vi "SP Perform Filter Skirt Limit Testing.vi"(0 "Filter Limit":T12={"Limit #"=1, "Parameter"={"Stimulus Port"=1, "Response Port"=2}, "Format"=enum."Lin Mag", "Filter Type"=enum."Bandpass", "Passband"={"Start/Center"=510.0, "Stop/Span"=610.0, "Units"=enum."MHz", "Freq Format"=enum."Start/Stop", "Bandwidth Attn"=3.0, "Passband Limit"=FALSE}, "Ripple"={"Ripple Limit"=TRUE, "Window On"=FALSE, "Ripple"=0.1, "Window"=10.0, "Units"=enum."MHz"}, "Attenuation Points"=[], "Skirt Points"=[{"Relative"=TRUE, "Connect"=FALSE, "Frequency"=500.0, "Units"=enum."MHz", "Attenuation"=4.0, "Relative Loss"=enum."Calculated Center", "Relative Freq"=1000.0}, {"Relative"=TRUE, "Connect"=TRUE, "Frequency"=509.0, "Units"=enum."MHz", "Attenuation"=4.0, "Relative Loss"=enum."Calculated Center", "Relative Freq"=1000.0}, {"Relative"=TRUE, "Connect"=FALSE, "Frequency"=611.0, "Units"=enum."MHz", "Attenuation"=4.0, "Relative Loss"=enum."Calculated Center", "Relative Freq"=1000.0}, {"Relative"=TRUE, "Connect"=TRUE, "Frequency"=620.0, "Units"=enum."MHz", "Attenuation"=4.0, "Relative Loss"=enum."Calculated Center", "Relative Freq"=1000.0}]} {"Parameter"."Stimulus Port" min=1 step=1; "Parameter"."Response Port" min=1 step=1; "Passband"."Bandwidth Attn" format="%.3g"; "Passband"."Stop/Span" format="%.3g"; "Passband"."Start/Center" format="%.3g"}, 5 "Data":T11={"F0"=500.0, "dF"=1.0, "Formatted Values"=[-6.0, -6.0, -6.0, -6.0, -6.0, -6.0, -5.0, -4.0, -3.0, -2.0, -1.0017226002993769, -0.8636286738753696, -1.012432061728755, -0.8135188671805874, -1.084383696215112, -1.192695586219516, -0.8228939725524264, -1.1588169801015764, -1.0069715761898415, -0.8118111488159718, -0.9516999033989667, -1.0842662636672022, -1.0261931083967077, -0.816874162233468, -0.8335770068326294, -1.1794529347576463, -1.1032959879886735, -1.197742447623333, -0.9631229100196212, -0.9908453124177325, -0.9835470980893588, -1.10217991844936, -0.8956607286257672, -0.8794782872077156, -0.9013683651609963, -1.0772188731817596, -0.992723355191172, -0.9536275499498994, -0.9874327685983141, -0.921963653527827, -0.8848787728556787, -1.1874980208218, -0.996957511881206, -0.9972503730309241, -0.8866139538542095, -1.07344181331393, -0.881559772443858, -1.0112449407130875, -0.9865384477979471, -0.9901446738263366, -1.1718630063784758, -0.9951725256878827, -0.931778781153855, -0.9846289731021831, -0.851763264124267, -0.9086965469391421, -0.8349429101974368, -0.8383742350256687, -1.106571816484691, -0.9554005266395742, -0.9376822403043366, -1.131287512516927, -1.0382288806403288, -0.917054052988136, -0.9489467877812984, -0.9264227759143271, -1.0918690925892351, -1.1668737446636852, -1.0021735712381068, -1.1541225361979714, -1.1931131329605709, -0.8730502330378824, -0.850411285659811, -1.137775166801135, -1.1870586525662095, -1.0926571181161528, -1.118993526927924, -1.1211410787283602, -0.8920697041785735, -0.888430731015914, -1.0656600076605476, -1.1666787859795846, -1.0713340188424678, -0.8625910088884297, -1.1434360227216422, -0.9217710376784376, -1.1218396445954617, -0.9558195687190933, -1.1773692443654946, -1.0827782751424972, -1.1567791336122029, -0.8684407402614696, -0.8177845157195978, -0.9040657051180614, -0.9313557288389804, -1.0236831450620423, -1.050426714979035, -0.8344777069605718, -0.8274082929927138, -1.1990080831766776, -1.0947798998491134, -1.1963114865246718, -1.0016247375583676, -1.0877110100652403, -1.1556028882288836, -1.1918380581525247, -0.9751292214691399, -0.8884133044813358, -1.0347444321214612, -0.9445125246491541, -2.0, -3.0, -4.0, -5.0, -6.0, -6.0, -6.0, -6.0, -6.0, -6.0]}, 9 "Generate Plot Output? (f)":bool, 11 "error in (no error)":errorcluster, 12 "Limit Results In":T2={"Limit #"=0, "Parameter"={"Stimulus Port"=1, "Response Port"=0}, "Bandwidth Pass?"={"Pass?"=FALSE, "Bandwidth"=0.0, "Limit"=0.0, "Units"=enum."Hz"}, "Ripple Pass?"={"Pass?"=FALSE, "Ripple"=0.0, "Limit"=0.0, "Format"=enum."Log Mag"}, "Attenuation Results"=[], "Skirt Results"=[], "Pass?"=FALSE} {"Parameter"."Stimulus Port" min=1 step=1; "Parameter"."Response Port" min=1 step=1}, 13 "Format":T1 caption="Display Format" items=["Log Mag", "Phase", "Expanded Phase", "Delay", "Smith", "Polar", "Lin Mag", "SWR", "Loss", "Real", "Imaginary"]) -> (1 "Upper Limits":cluster{"x values":dbl[], "y values":dbl[]}[](array[cluster]), 3 "Lower Limits":cluster{"x values":dbl[], "y values":dbl[]}[](array[cluster]), 4 "Limits Pass/Fail":cluster{"Upper Pass?":bool, "Lower Pass?":bool}, 6 "Upper and Lower Limits":T10={"Upper Limit"={"F0"=500.0, "dF"=1.0, "Formatted Values"=[-6.0, -6.0, -6.0, -6.0, -6.0, -6.0, -5.0, -4.0, -3.0, -2.0, -1.0017226002993769, -0.8636286738753696, -1.012432061728755, -0.8135188671805874, -1.084383696215112, -1.192695586219516, -0.8228939725524264, -1.1588169801015764, -1.0069715761898415, -0.8118111488159718, -0.9516999033989667, -1.0842662636672022, -1.0261931083967077, -0.816874162233468, -0.8335770068326294, -1.1794529347576463, -1.1032959879886735, -1.197742447623333, -0.9631229100196212, -0.9908453124177325, -0.9835470980893588, -1.10217991844936, -0.8956607286257672, -0.8794782872077156, -0.9013683651609963, -1.0772188731817596, -0.992723355191172, -0.9536275499498994, -0.9874327685983141, -0.921963653527827, -0.8848787728556787, -1.1874980208218, -0.996957511881206, -0.9972503730309241, -0.8866139538542095, -1.07344181331393, -0.881559772443858, -1.0112449407130875, -0.9865384477979471, -0.9901446738263366, -1.1718630063784758, -0.9951725256878827, -0.931778781153855, -0.9846289731021831, -0.851763264124267, -0.9086965469391421, -0.8349429101974368, -0.8383742350256687, -1.106571816484691, -0.9554005266395742, -0.9376822403043366, -1.131287512516927, -1.0382288806403288, -0.917054052988136, -0.9489467877812984, -0.9264227759143271, -1.0918690925892351, -1.1668737446636852, -1.0021735712381068, -1.1541225361979714, -1.1931131329605709, -0.8730502330378824, -0.850411285659811, -1.137775166801135, -1.1870586525662095, -1.0926571181161528, -1.118993526927924, -1.1211410787283602, -0.8920697041785735, -0.888430731015914, -1.0656600076605476, -1.1666787859795846, -1.0713340188424678, -0.8625910088884297, -1.1434360227216422, -0.9217710376784376, -1.1218396445954617, -0.9558195687190933, -1.1773692443654946, -1.0827782751424972, -1.1567791336122029, -0.8684407402614696, -0.8177845157195978, -0.9040657051180614, -0.9313557288389804, -1.0236831450620423, -1.050426714979035, -0.8344777069605718, -0.8274082929927138, -1.1990080831766776, -1.0947798998491134, -1.1963114865246718, -1.0016247375583676, -1.0877110100652403, -1.1556028882288836, -1.1918380581525247, -0.9751292214691399, -0.8884133044813358, -1.0347444321214612, -0.9445125246491541, -2.0, -3.0, -4.0, -5.0, -6.0, -6.0, -6.0, -6.0, -6.0, -6.0]}, "Lower Limit"={"F0"=500.0, "dF"=1.0, "Formatted Values"=[-6.0, -6.0, -6.0, -6.0, -6.0, -6.0, -5.0, -4.0, -3.0, -2.0, -1.0017226002993769, -0.8636286738753696, -1.012432061728755, -0.8135188671805874, -1.084383696215112, -1.192695586219516, -0.8228939725524264, -1.1588169801015764, -1.0069715761898415, -0.8118111488159718, -0.9516999033989667, -1.0842662636672022, -1.0261931083967077, -0.816874162233468, -0.8335770068326294, -1.1794529347576463, -1.1032959879886735, -1.197742447623333, -0.9631229100196212, -0.9908453124177325, -0.9835470980893588, -1.10217991844936, -0.8956607286257672, -0.8794782872077156, -0.9013683651609963, -1.0772188731817596, -0.992723355191172, -0.9536275499498994, -0.9874327685983141, -0.921963653527827, -0.8848787728556787, -1.1874980208218, -0.996957511881206, -0.9972503730309241, -0.8866139538542095, -1.07344181331393, -0.881559772443858, -1.0112449407130875, -0.9865384477979471, -0.9901446738263366, -1.1718630063784758, -0.9951725256878827, -0.931778781153855, -0.9846289731021831, -0.851763264124267, -0.9086965469391421, -0.8349429101974368, -0.8383742350256687, -1.106571816484691, -0.9554005266395742, -0.9376822403043366, -1.131287512516927, -1.0382288806403288, -0.917054052988136, -0.9489467877812984, -0.9264227759143271, -1.0918690925892351, -1.1668737446636852, -1.0021735712381068, -1.1541225361979714, -1.1931131329605709, -0.8730502330378824, -0.850411285659811, -1.137775166801135, -1.1870586525662095, -1.0926571181161528, -1.118993526927924, -1.1211410787283602, -0.8920697041785735, -0.888430731015914, -1.0656600076605476, -1.1666787859795846, -1.0713340188424678, -0.8625910088884297, -1.1434360227216422, -0.9217710376784376, -1.1218396445954617, -0.9558195687190933, -1.1773692443654946, -1.0827782751424972, -1.1567791336122029, -0.8684407402614696, -0.8177845157195978, -0.9040657051180614, -0.9313557288389804, -1.0236831450620423, -1.050426714979035, -0.8344777069605718, -0.8274082929927138, -1.1990080831766776, -1.0947798998491134, -1.1963114865246718, -1.0016247375583676, -1.0877110100652403, -1.1556028882288836, -1.1918380581525247, -0.9751292214691399, -0.8884133044813358, -1.0347444321214612, -0.9445125246491541, -2.0, -3.0, -4.0, -5.0, -6.0, -6.0, -6.0, -6.0, -6.0, -6.0]}}, 10 "Failures":cluster{"x values":dbl[], "y values":dbl[]}[](array[cluster]), 14 "Limit Results Out":T2={"Limit #"=0, "Parameter"={"Stimulus Port"=1, "Response Port"=0}, "Bandwidth Pass?"={"Pass?"=FALSE, "Bandwidth"=0.0, "Limit"=0.0, "Units"=enum."Hz"}, "Ripple Pass?"={"Pass?"=FALSE, "Ripple"=0.0, "Limit"=0.0, "Format"=enum."Log Mag"}, "Attenuation Results"=[], "Skirt Results"=[], "Pass?"=FALSE} {"Parameter"."Stimulus Port" min=1 step=1; "Parameter"."Response Port" min=1 step=1}, 15 "error out":errorcluster)   [LabVIEW 2011]
uses:
  TypeDefs/SP Filter.ctl
  TypeDefs/SP Parameter.ctl
  TypeDefs/SP Format.ctl
  TypeDefs/SP Filter Type.ctl
  TypeDefs/SP Filter Passband.ctl
  TypeDefs/SP Frequency Units.ctl
  TypeDefs/SP Frequency Format.ctl
  TypeDefs/SP Filter Ripple.ctl
  TypeDefs/SP Attenuation Point.ctl
  TypeDefs/SP Attenuation Type.ctl
  TypeDefs/SP Skirt Rejection Point.ctl
  TypeDefs/SP Relative Loss.ctl
  TypeDefs/SP Limit Results.ctl
  TypeDefs/SP Bandwidth Limit Results.ctl
  TypeDefs/SP Ripple Limit Results.ctl
  TypeDefs/SP Attenuation Limit Results.ctl
  TypeDefs/SP Skirt Limit Results.ctl
  TypeDefs/SP Display Format.ctl
  <vilib>/Analysis/NI_AALBase.lvlib
panel:
  out "Plot Output":cluster{"x values":dbl[], "y values":dbl[]}[](graph)
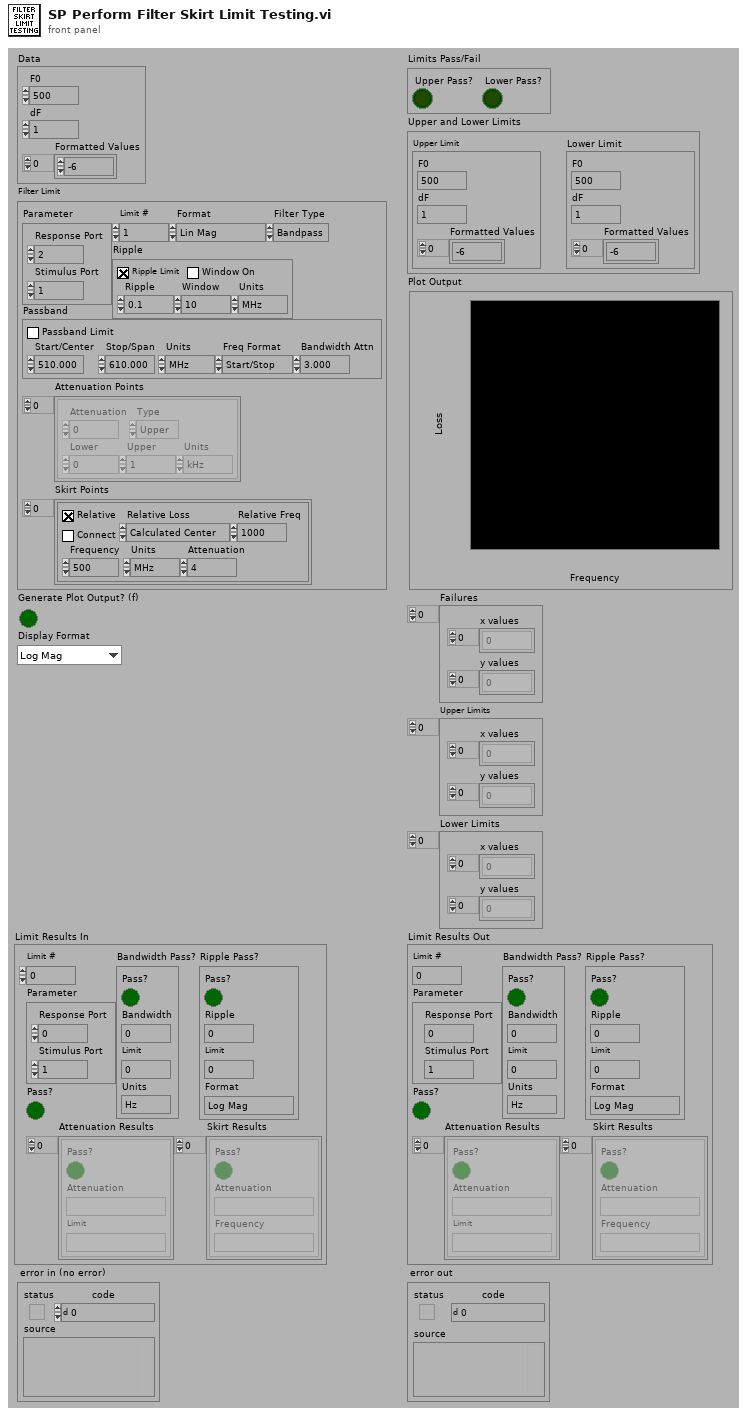
[diagram p1: front panel]
types:
  T1 = typedef "SP Display Format.ctl" = i32
  T2 = typedef "SP Limit Results.ctl" = cluster{"Limit #":i8, "Parameter":T3, "Bandwidth Pass?":T4, "Ripple Pass?":T6, "Attenuation Results":T8[], "Skirt Results":T9[], "Pass?":bool}
  T3 = typedef "SP Parameter.ctl" = cluster{"Stimulus Port":i8, "Response Port":i8}
  T4 = typedef "SP Bandwidth Limit Results.ctl" = cluster{"Pass?":bool, "Bandwidth":dbl, "Limit":dbl, "Units":T5}
  T5 = typedef "SP Frequency Units.ctl" = enum16{"Hz", "kHz", "MHz", "GHz", "Points"}
  T6 = typedef "SP Ripple Limit Results.ctl" = cluster{"Pass?":bool, "Ripple":dbl, "Limit":dbl, "Format":T7}
  T7 = typedef "SP Format.ctl" = enum16{"Log Mag", "Lin Mag", "SWR", "Phase", "Expanded Phase", "Delay", "Insertion Loss", "Isolation", "Return Loss"}
  T8 = typedef "SP Attenuation Limit Results.ctl" = cluster{"Pass?":bool, "Attenuation":string, "Limit":string}
  T9 = typedef "SP Skirt Limit Results.ctl" = cluster{"Pass?":bool, "Attenuation":string, "Frequency":string}
  T10 = cluster{"Upper Limit":cluster{"F0":dbl, "dF":dbl, "Formatted Values":dbl[]}, "Lower Limit":cluster{"F0":dbl, "dF":dbl, "Formatted Values":dbl[]}}
  T11 = cluster{"F0":dbl, "dF":dbl, "Formatted Values":dbl[]}
  T12 = typedef "SP Filter.ctl" = cluster{"Limit #":i8, "Parameter":T3, "Format":T7, "Filter Type":T13, "Passband":T14, "Ripple":T16, "Attenuation Points":T17[], "Skirt Points":T19[]}
  T13 = typedef "SP Filter Type.ctl" = enum16{"Lowpass", "Highpass", "Bandpass", "Bandstop"}
  T14 = typedef "SP Filter Passband.ctl" = cluster{"Start/Center":dbl, "Stop/Span":dbl, "Units":T5, "Freq Format":T15, "Bandwidth Attn":dbl, "Passband Limit":bool}
  T15 = typedef "SP Frequency Format.ctl" = enum16{"Start/Stop", "Center/Span"}
  T16 = typedef "SP Filter Ripple.ctl" = cluster{"Ripple Limit":bool, "Window On":bool, "Ripple":dbl, "Window":dbl, "Units":T5}
  T17 = typedef "SP Attenuation Point.ctl" = cluster{"Attenuation":dbl, "Type":T18, "Lower":dbl, "Upper":dbl, "Units":T5}
  T18 = typedef "SP Attenuation Type.ctl" = enum16{"Center", "Lower", "Upper"}
  T19 = typedef "SP Skirt Rejection Point.ctl" = cluster{"Relative":bool, "Connect":bool, "Frequency":dbl, "Units":T5, "Attenuation":dbl, "Relative Loss":T20, "Relative Freq":dbl}
  T20 = typedef "SP Relative Loss.ctl" = enum16{"Calculated Center", "Passband Minimum", "Passband Maximum", "Passband Average", "Frequency"}
  T21 = cluster{"x0":dbl, "dx":dbl, "Stored Values":dbl[]}
  T22 = cluster{"Limit":cluster{"x0":dbl, "dx":dbl, "Y":dbl[]}, "Limit":cluster{"x0":dbl, "dx":dbl, "Stored Values":dbl[]}}
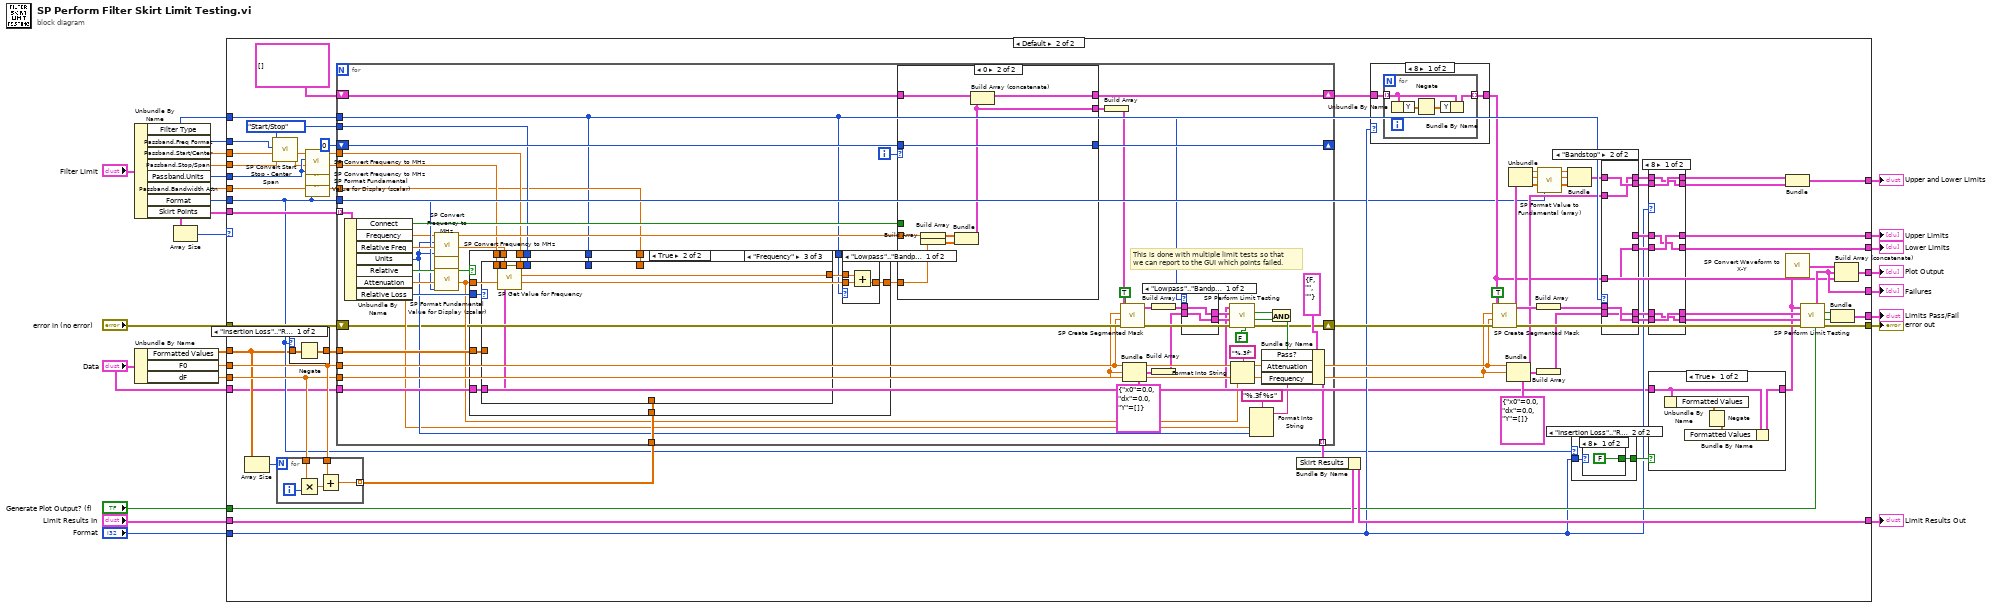
[diagram p0: block diagram]
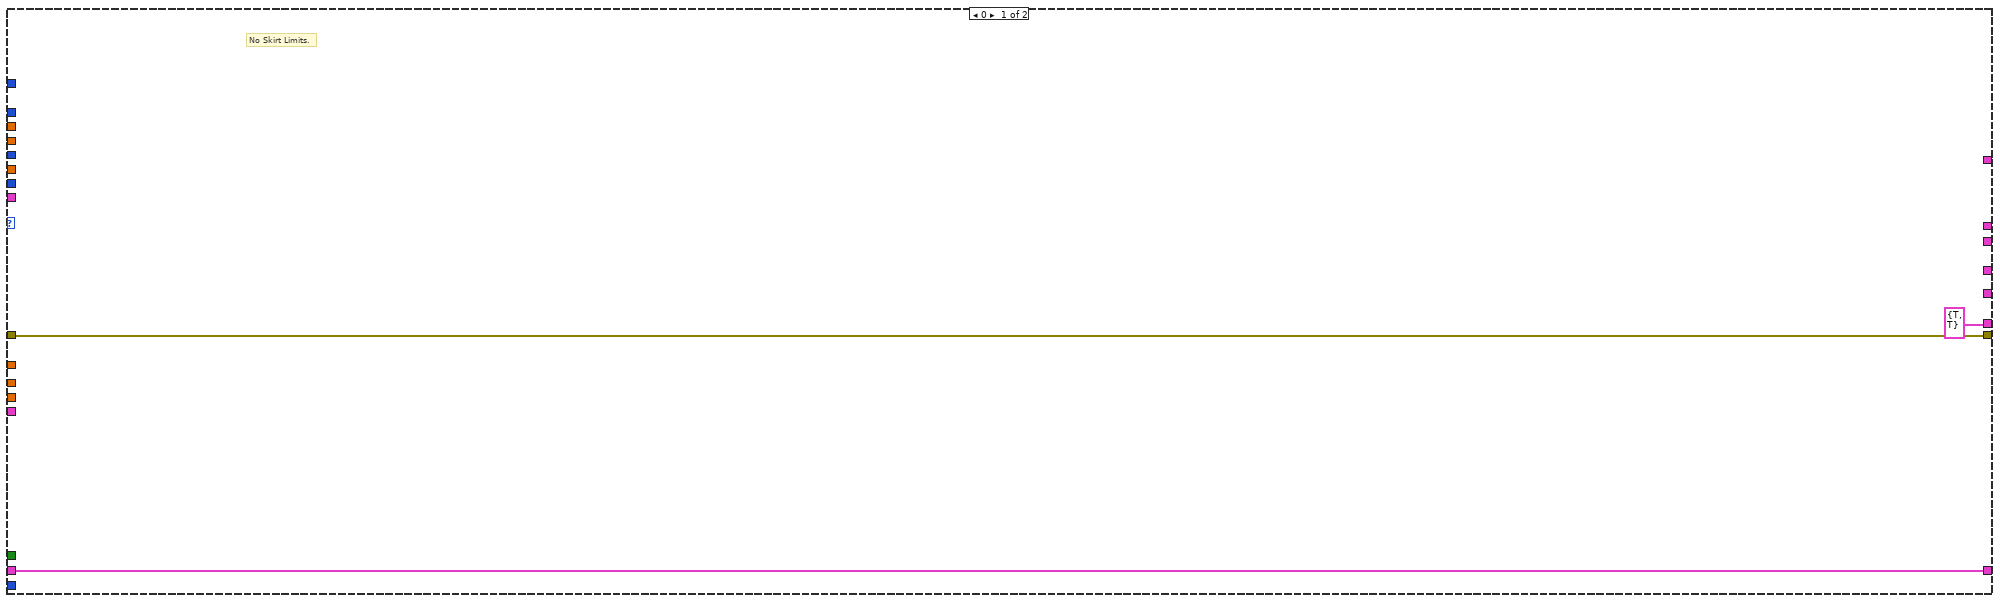
[diagram p2: hidden frame]
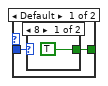
[diagram p4: hidden frame]
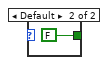
[diagram p5: hidden frame]
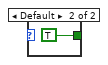
[diagram p6: hidden frame]
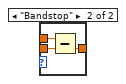
[diagram p13: hidden frame]
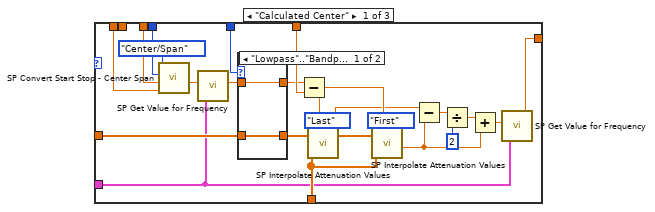
[diagram p14: hidden frame]
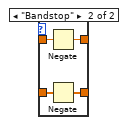
[diagram p15: hidden frame]
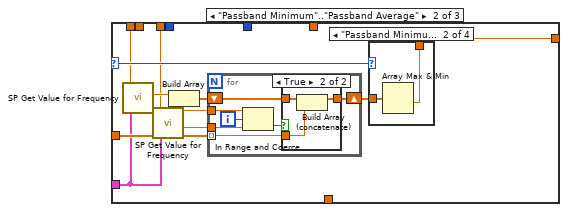
[diagram p16: hidden frame]
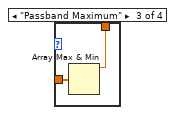
[diagram p18: hidden frame]
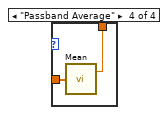
[diagram p19: hidden frame]
diagram:
  n1 = Unbundle By Name("Filter Limit") -> ("Filter Type"=w17:T13, "Passband.Freq Format"=w16:T15, "Passband.Start/Center"=w25:dbl, "Passband.Stop/Span"=w24:dbl, "Passband.Units"=w23:T5, "Passband.Bandwidth Attn"=w12:dbl, "Format"=w13:T7, "Skirt Points"=w14:T19[])
  n2 = Unbundle By Name("Data") -> ("Formatted Values"=w22:dbl[], "F0"=w11:dbl, "dF"=w10:dbl)
  n3 = Array Size(array=w14) -> (size(s)=w15:i32)
  n4 = case shown="Default" w15 {
    tunnel: w17 -> [_ w76]
    tunnel: w25 -> [_ w90]
    tunnel: w24 -> [_ w89]
    tunnel: w23 -> [_ w95]
    tunnel: w22 -> [_ w32]
    tunnel: "Data" -> [_ w31]
    tunnel: "Generate Plot Output? (f)" -> [_ w67]
    tunnel: "error in (no error)" -> [w29 w71]
    tunnel: [w29 w92] -> w18
    tunnel: w16 -> [_ w86]
    tunnel: w14 -> [_ w85]
    tunnel: w13 -> [_ w33]
    tunnel: w12 -> [_ w82]
    tunnel: w11 -> [_ w64]
    tunnel: w10 -> [_ w63]
    tunnel: [_ w74] -> w9
    tunnel: [_ w66] -> w8
    tunnel: [_ w37] -> w7
    tunnel: [_ w30] -> w6
    tunnel: "Limit Results In" -> [w28 w70]
    tunnel: [w28 w69] -> w4
    tunnel: [cluster{"Upper Pass?":bool, "Lower Pass?":bool} {"Upper Pass?"=TRUE, "Lower Pass?"=TRUE} w59] -> w3
    tunnel: [_ w51] -> w2
    tunnel: "Format" -> [_ w34]
    frame 0 {
      # "No Skirt Limits."
    }
    frame Default {
      w83 = SP_Frequency_Format."Start/Stop" ("Freq Format To")
      n5 = Array Size(array=w32) -> (size(s)=w80:i32)
      n6 = call "SP Convert Start Stop - Center Span.vi"("Stop/Span In"=w89, "Start/Center In"=w90, "Freq Format From"=w86, "Freq Format To"=w83) -> ("Stop/Span Out"=w88:dbl, "Start/Center Out"=w87:dbl)  [unwired: 6 out]
      n7 = for {
        N: w80 -> [_]
        tunnel: w63 -> [w144]
        tunnel: w64 -> [w142]
        tunnel: [w141] -> w79 mode=indexing
        i -> [w145]
        n8 = Multiply(x=w144, y=w145) -> (x*y=w143:dbl)
        n9 = Add(x=w142, y=w143) -> (x+y=w141:dbl)
      }
      n10 = case shown="\"Insertion Loss\"..\"Return Loss\"" w33 {
        tunnel: w32 -> [w129 w130]
        tunnel: [w128 w130] -> w50
        frame "Insertion Loss".."Return Loss" {
          n11 = Negate(x=w129) -> (-x=w128:dbl[])
        }
        frame Default {
        }
      }
      n12 = call "SP Convert Frequency to MHz.vi"("Units"=w95, "Frequency"=w87) -> ("Converted Frequency"=w93:dbl)  [unwired: 1 in, 8 out]
      n13 = call "SP Convert Frequency to MHz.vi"("Units"=w95, "Frequency"=w88) -> ("Converted Frequency"=w94:dbl)  [unwired: 1 in, 8 out]
      n14 = call "SP Format Fundamental Value for Display (scalar).vi"("Format"=w33, "Stored Value (0, linear)"=w82) -> ("Display Value"=w81:dbl)  [unwired: 5 out]
      n15 = for {
        tunnel: w94 -> [w181]
        tunnel: w93 -> [w182]
        tunnel: w85 -> [w196] mode=indexing
        shift-right: [w193] -> w49
        shift-left: cluster{"X":dbl[], "Y":dbl[]}[] [] ("Limit Specification") -> [w194]
        shift-right: [w192] -> _
        shift-left: 0 -> [w191]
        tunnel: w33 -> [w184]
        tunnel: w83 -> [w179]
        tunnel: w81 -> [w178]
        tunnel: w76 -> [w155]
        tunnel: w50 -> [w177]
        tunnel: w31 -> [w156]
        tunnel: w79 -> [w176]
        shift-right: [w151] -> w72
        shift-left: w71 -> [w158]
        tunnel: w64 -> [w149]
        tunnel: w63 -> [w148]
        tunnel: [w174] -> w68 mode=indexing
        i -> [w195]
        # "This is done with multiple limit tests so that\nwe can report to the GUI which points failed."
        n16 = Unbundle By Name(w196) -> ("Connect"=w188:bool, "Frequency"=w169:dbl, "Relative Freq"=w189:dbl, "Units"=w170:T5, "Relative"=w186:bool, "Attenuation"=w187:dbl, "Relative Loss"=w183:T20)
        n17 = call "SP Convert Frequency to MHz.vi"("Units"=w170, "Frequency"=w169) -> ("Converted Frequency"=w190:dbl)  [unwired: 1 in, 8 out]
        n18 = call "SP Convert Frequency to MHz.vi"("Units"=w170, "Frequency"=w189) -> ("Converted Frequency"=w180:dbl)  [unwired: 1 in, 8 out]
        n19 = call "SP Format Fundamental Value for Display (scalar).vi"("Format"=w184, "Stored Value (0, linear)"=w187) -> ("Display Value"=w172:dbl)  [unwired: 5 out]
        n20 = case shown="True" w186 {
          tunnel: w172 -> [w201 w209]
          tunnel: [w201 w208] -> w185
          tunnel: w183 -> [_ w215]
          tunnel: w182 -> [_ w214]
          tunnel: w181 -> [_ w213]
          tunnel: w177 -> [_ w212]
          tunnel: w180 -> [_ w211]
          tunnel: w179 -> [_ w207]
          tunnel: w156 -> [_ w206]
          tunnel: w155 -> [_ w205]
          tunnel: w178 -> [_ w204]
          tunnel: w176 -> [_ w203]
          tunnel: w155 -> [_ w202]
          frame False {
          }
          frame True {
            n21 = case shown="\"Frequency\"" w215 {
              selector: w215 -> [_ w258 _]
              tunnel: w214 -> [w242 w254 _]
              tunnel: w213 -> [w243 w256 _]
              tunnel: w212 -> [w232 w261 _]
              tunnel: [w224 w259 w281] -> w210
              tunnel: w211 -> [_ _ w282]
              tunnel: w207 -> [w241 _ _]
              tunnel: w206 -> [w226 w251 w280]
              tunnel: w205 -> [w234 _ _]
              tunnel: w204 -> [w223 _ _]
              tunnel: w203 -> [w239 _ _]
              frame "Calculated Center" {
                n22 = call "SP Convert Start Stop - Center Span.vi"("Stop/Span In"=w243, "Start/Center In"=w242, "Freq Format From"=w241, "Freq Format To"=SP_Frequency_Format."Center/Span") -> ("Start/Center Out"=w240:dbl)  [unwired: 7 out]
                n23 = call "SP Get Value for Frequency.vi"("Data"=w226, "Frequency (MHz)"=w240) -> ("Value"=w233:dbl)  [unwired: 5 out]
                n24 = case shown="\"Lowpass\"..\"Bandpass\"" w234 {
                  tunnel: w233 -> [w245 w250]
                  tunnel: w232 -> [w246 w248]
                  tunnel: [w246 w247] -> w231
                  tunnel: [w245 w249] -> w222
                  frame "Lowpass".."Bandpass" {
                  }
                  frame "Bandstop" {
                    n25 = Negate(x=w250) -> (-x=w249:dbl)
                    n26 = Negate(x=w248) -> (-x=w247:dbl[])
                  }
                }
                n27 = Subtract(x=w222, y=w223) -> (x-y=w236:dbl)
                n28 = call "SP Interpolate Attenuation Values.vi"("Instance (First)"=enum16{"First", "Last"}."Last", "Attenuation Value"=w236, "X Values"=w239, "Y Values"=w231) -> ("Interpolated X Value"=w235:dbl)  [unwired: 7 out]
                n29 = call "SP Interpolate Attenuation Values.vi"("Instance (First)"=enum16{"First", "Last"}."First", "Attenuation Value"=w236, "X Values"=w239, "Y Values"=w231) -> ("Interpolated X Value"=w227:dbl)  [unwired: 7 out]
                n30 = Subtract(x=w235, y=w227) -> (x-y=w229:dbl)
                n31 = Divide(x=w229, y=i8 2) -> (x/y=w230:dbl)
                n32 = Add(x=w230, y=w227) -> (x+y=w225:dbl)
                n33 = call "SP Get Value for Frequency.vi"("Data"=w226, "Frequency (MHz)"=w225) -> ("Value"=w224:dbl)  [unwired: 5 out]
              }
              frame "Passband Minimum".."Passband Average" {
                n34 = call "SP Get Value for Frequency.vi"("Data"=w251, "Frequency (MHz)"=w256) -> ("Fractional Index"=w255:dbl, "Value"=w257:dbl)  [unwired: 4 out]
                n35 = call "SP Get Value for Frequency.vi"("Data"=w251, "Frequency (MHz)"=w254) -> ("Fractional Index"=w252:dbl, "Value"=w253:dbl)  [unwired: 4 out]
                n36 = Build Array(w257, w253) -> (w262:dbl[])
                n37 = for {
                  shift-right: [w271] -> w260
                  shift-left: w262 -> [w275]
                  tunnel: w261 -> [w272] mode=indexing
                  tunnel: w255 -> [w270]
                  tunnel: w252 -> [w269]
                  i -> [w274]
                  n38 = In Range and Coerce(upper limit=w270, x=w274, lower limit=w269) -> (In Range?=w273:bool)  [unwired: 1 out]
                  n39 = case shown="True" w273 {
                    tunnel: w275 -> [w276 w279]
                    tunnel: w272 -> [_ w278]
                    tunnel: [w276 w277] -> w271
                    frame False {
                    }
                    frame True {
                      n40 = Build Array (concatenate)(w279, w278) -> (w277:dbl[])
                    }
                  }
                }
                n41 = case shown="\"Passband Minimum\"" w258 {
                  tunnel: w260 -> [_ w264 w266 w268]
                  tunnel: [_ w263 w265 w267] -> w259
                  frame Default {
                  }
                  frame "Passband Minimum" {
                    n42 = Array Max & Min(array=w264) -> (min value=w263:dbl)  [unwired: 3 out]
                  }
                  frame "Passband Maximum" {
                    n43 = Array Max & Min(array=w266) -> (max value=w265:dbl)  [unwired: 3 out]
                  }
                  frame "Passband Average" {
                    n44 = call <vilib>:"Mean.vi"("X"=w268) -> ("mean"=w267:dbl)  [unwired: 1 out]
                  }
                }
              }
              frame "Frequency" {
                n45 = call "SP Get Value for Frequency.vi"("Data"=w280, "Frequency (MHz)"=w282) -> ("Value"=w281:dbl)  [unwired: 5 out]
              }
            }
            n46 = case shown="\"Lowpass\"..\"Bandpass\"" w202 {
              tunnel: w210 -> [w218 w221]
              tunnel: w209 -> [w217 w220]
              tunnel: [w216 w219] -> w208
              frame "Lowpass".."Bandpass" {
                n47 = Add(x=w218, y=w217) -> (x+y=w216:dbl)
              }
              frame "Bandstop" {
                n48 = Subtract(x=w221, y=w220) -> (x-y=w219:dbl)
              }
            }
          }
        }
        n49 = case shown="0" w195 {
          tunnel: w194 -> [w290 w318]
          tunnel: [w289 w317] -> w193
          tunnel: [w287 w312] -> w192
          tunnel: w191 -> [w288 w312]
          tunnel: w190 -> [w285 w316]
          tunnel: w188 -> [w286 _]
          tunnel: w185 -> [w284 w315]
          tunnel: [w283 w311] -> w154
          frame Default {
            n50 = case shown="False" w286 {
              tunnel: w285 -> [w295 w307]
              tunnel: w284 -> [w292 w306]
              tunnel: w288 -> [w297 w302]
              tunnel: w290 -> [w299 w303]
              tunnel: [w296 w302] -> w287
              tunnel: [w298 w301] -> w289
              tunnel: [w291 w300] -> w283
              frame False {
                # "Start a new limit segment..."
                n51 = Build Array(w295) -> (w294:dbl[])
                n52 = Build Array(w292) -> (w293:dbl[])
                n53 = Increment(x=w297) -> (x+1=w296:i32)
                n54 = Bundle(w294, w293) -> (w291:cluster{dbl[], dbl[]})  [unwired: 1 out]
                n55 = Build Array (concatenate)(w299, w291) -> (w298:cluster{"X":dbl[], "Y":dbl[]}[])
              }
              frame True {
                n56 = Index Array(array=w303, index=w302) -> (element=w310:cluster{"X":dbl[], "Y":dbl[]})
                n57 = Unbundle(w310) -> ("X"=w309:dbl[], "Y"=w308:dbl[])
                n58 = Build Array (concatenate)(w309, w307) -> (w305:dbl[])
                n59 = Build Array (concatenate)(w308, w306) -> (w304:dbl[])
                n60 = Bundle(w305, w304) -> (w300:cluster{dbl[], dbl[]})  [unwired: 1 out]
                n61 = Replace Array Subset(array=w303, new element=w300, index=w302) -> (w301:cluster{"X":dbl[], "Y":dbl[]}[])
              }
            }
          }
          frame 0 {
            n62 = Build Array(w316) -> (w314:dbl[])
            n63 = Build Array(w315) -> (w313:dbl[])
            n64 = Bundle(w314, w313) -> (w311:cluster{dbl[], dbl[]})  [unwired: 1 out]
            n65 = Build Array (concatenate)(w318, w311) -> (w317:cluster{"X":dbl[], "Y":dbl[]}[])
          }
        }
        n66 = Build Array(w154) -> (w153:cluster{dbl[], dbl[]}[])
        n67 = call "SP Create Segmented Mask.vi"("Reset"=TRUE, "error in"=w158, "x0"=w149, "dx"=w148, "Specification Cluster"=w153) -> ("error out"=w162:errorcluster, "Limit"=w159:cluster{"x0":dbl, "dx":dbl, "Y":dbl[]})  [unwired: 3 out]
        n68 = Bundle(cluster=cluster{"x0":dbl, "dx":dbl, "Y":dbl[]} {"x0"=0.0, "dx"=0.0, "Y"=[]} ("Limit"), "x0"=w149, "dx"=w148) -> (w147:cluster{"x0":dbl, "dx":dbl, "Y":dbl[]})  [unwired: 1 out]
        n69 = Build Array(w159) -> (w161:cluster{"x0":dbl, "dx":dbl, "Y":dbl[]}[])
        n70 = Build Array(w147) -> (w146:cluster{"x0":dbl, "dx":dbl, "Y":dbl[]}[])
        n71 = case shown="\"Lowpass\"..\"Bandpass\"" w155 {
          tunnel: w161 -> [w198 w200]
          tunnel: [w198 w199] -> w163
          tunnel: [w197 w200] -> w164
          tunnel: w146 -> [w197 w199]
          frame "Lowpass".."Bandpass" {
          }
          frame "Bandstop" {
          }
        }
        n72 = call "SP Perform Limit Testing.vi"("Generate Plot Output? (f)"=FALSE, "error in (no error)"=w162, "LLimits"=w164, "ULimits"=w163, "Data"=w156) -> ("error out"=w151:errorcluster, "Lower Pass?"=w166:bool, "Upper Pass?"=w165:bool)  [unwired: 2 in, 2 out]
        n73 = Format Into String(format string="%.3f", w172) -> (resulting string=w168:string)  [unwired: 2 in, 1 out]
        n74 = Format Into String(format string="%.3f %s", w169, w170) -> (resulting string=w167:string)  [unwired: 2 in, 1 out]
        n75 = And(x=w165, y=w166) -> (x .and. y?=w157:bool)
        n76 = Bundle By Name(cluster=T9 {"Pass?"=FALSE, "Attenuation"="", "Frequency"=""} ("Skirt Results"), "Pass?"=w157, "Attenuation"=w168, "Frequency"=w167) -> (w174:T9)
      }
      n77 = Bundle By Name(cluster=w70, "Skirt Results"=w68) -> (w69:T2)
      n78 = case shown="8" w34 {
        tunnel: w49 -> [w122 w127]
        tunnel: [w121 w127] -> w48
        frame 8 {
          n79 = for {
            tunnel: w122 -> [w126] mode=indexing
            tunnel: [w125] -> w121 mode=indexing
            n80 = Unbundle By Name(w126) -> ("Y"=w124:dbl[])
            n81 = Negate(x=w124) -> (-x=w123:dbl[])
            n82 = Bundle By Name(cluster=w126, "Y"=w123) -> (w125:cluster{"X":dbl[], "Y":dbl[]})
          }
        }
        frame Default {
        }
      }
      n83 = call "SP Create Segmented Mask.vi"("Reset"=TRUE, "error in"=w72, "x0"=w64, "dx"=w63, "Specification Cluster"=w48) -> ("error out"=w78:errorcluster, "Limit"=w54:cluster{"x0":dbl, "dx":dbl, "Y":dbl[]})  [unwired: 3 out]
      n84 = Bundle(cluster=cluster{"x0":dbl, "dx":dbl, "Y":dbl[]} {"x0"=0.0, "dx"=0.0, "Y"=[]} ("Limit"), "x0"=w64, "dx"=w63) -> (w52:cluster{"x0":dbl, "dx":dbl, "Y":dbl[]})  [unwired: 1 out]
      n85 = Unbundle(w54) -> ("x0"=w58:dbl, "dx"=w57:dbl, "Y"=w56:dbl[])
      n86 = Build Array(w54) -> (w77:cluster{"x0":dbl, "dx":dbl, "Y":dbl[]}[])
      n87 = Build Array(w52) -> (w62:cluster{"x0":dbl, "dx":dbl, "Y":dbl[]}[])
      n88 = call "SP Format Value to Fundamental (array).vi"("Sxx Display Format"=w33, "Display Values"=w56) -> ("Stored Values"=w55:dbl[])  [unwired: 5 out]
      n89 = Bundle("x0"=w58, "dx"=w57, "Stored Values"=w55) -> (w53:T21)  [unwired: 1 out]
      n90 = case shown="\"Insertion Loss\"..\"Return Loss\"" w33 {
        tunnel: [w102 w106] -> w36
        tunnel: w34 -> [w101 w105]
        frame Default {
          n91 = case shown="8" w101 {
            tunnel: [TRUE FALSE] -> w102
            frame 8 {
            }
            frame Default {
            }
          }
        }
        frame "Insertion Loss".."Return Loss" {
          n92 = case shown="8" w105 {
            tunnel: [FALSE TRUE] -> w106
            frame 8 {
            }
            frame Default {
            }
          }
        }
      }
      n93 = case shown="\"Bandstop\"" w76 {
        tunnel: w77 -> [w135 w140]
        tunnel: [w135 w138] -> w47
        tunnel: [w133 w140] -> w46
        tunnel: w48 -> [w134 w139]
        tunnel: [_ w139] -> w44
        tunnel: [w134 _] -> w45
        tunnel: w62 -> [w133 w138]
        tunnel: w53 -> [w132 w137]
        tunnel: [w132 w136] -> w42
        tunnel: [w131 w137] -> w43
        tunnel: w52 -> [w131 w136]
        frame "Lowpass".."Bandpass" {
        }
        frame "Bandstop" {
        }
      }
      n94 = case shown="8" w34 {
        tunnel: w47 -> [w110 w117]
        tunnel: w46 -> [w111 w118]
        tunnel: w45 -> [w109 w115]
        tunnel: w44 -> [w112 w116]
        tunnel: w43 -> [w114 w120]
        tunnel: w42 -> [w113 w119]
        tunnel: [w113 w120] -> w41
        tunnel: [w114 w119] -> w40
        tunnel: [w110 w118] -> w39
        tunnel: [w111 w117] -> w38
        tunnel: [w109 w116] -> w37
        tunnel: [w112 w115] -> w30
        frame 8 {
        }
        frame Default {
        }
      }
      n95 = case shown="True" w36 {
        tunnel: w31 -> [w99 w100]
        tunnel: [w98 w100] -> w35
        frame True {
          n96 = Unbundle By Name(w99) -> ("Formatted Values"=w97:dbl[])
          n97 = Negate(x=w97) -> (-x=w96:dbl[])
          n98 = Bundle By Name(cluster=w99, "Formatted Values"=w96) -> (w98:T11)
        }
        frame False {
        }
      }
      n99 = Bundle("Limit"=w40, "Limit"=w41) -> (w51:T22)  [unwired: 1 out]
      n100 = call "SP Convert Waveform to X-Y.vi"("Waveform"=w35) -> ("X-Y"=w75:cluster{"X":dbl[], "Y":dbl[]})
      n101 = call "SP Perform Limit Testing.vi"("Generate Plot Output? (f)"=w67, "error in (no error)"=w78, "LLimits"=w39, "ULimits"=w38, "Data"=w35) -> ("error out"=w92:errorcluster, "Lower Pass?"=w60:bool, "Upper Pass?"=w61:bool, "Failures"=w66:cluster{"x values":dbl[], "y values":dbl[]}[])  [unwired: 2 in, 1 out]
      n102 = Bundle("Upper Pass?"=w61, "Lower Pass?"=w60) -> (w59:cluster{"Upper Pass?":bool, "Lower Pass?":bool})  [unwired: 1 out]
      n103 = Build Array (concatenate)(w75, w66, w48) -> (w74:cluster{"X":dbl[], "Y":dbl[]}[])
    }
  }
  "Limits Pass/Fail" <- w3
  "Upper and Lower Limits" <- w2
  "Plot Output" <- w9
  "error out" <- w18
  "Upper Limits" <- w6
  "Lower Limits" <- w7
  "Failures" <- w8
  "Limit Results Out" <- w4
